vi "Feeder_Begin.vi"   [LabVIEW 2020]
uses:
  Subsystems/Magazine/Magazine_Cluster.ctl
  Subsystems/Magazine/Magazine_Control_States.ctl
  Subsystems/Intake/Intake_cluster.ctl
  Subsystems/Intake/Intake_control_states.ctl
  Subsystems/Funnel/Funnel_Cluster.ctl
  Subsystems/Funnel/Control_States_Funnel.ctl
  Feeder_Cluster.ctl
  Feeder_Control_States.ctl
  Globals/Magazine_Globals.vi
  Globals/Intake_Globals.vi
  Globals/Funnel_global.vi
  Globals/Feeder_Globals.vi
types:
  T1 = typedef "Feeder_Cluster.ctl" = cluster{"Firing":bool, "Load":bool, "Magazine_%Vbus":dbl, "Funnel_%Vbus":dbl, "Intake_%Vbus":dbl, "Manual_Extend":bool, "Outtake":bool, "Parameters":dbl[], "Auto_Notifier":refnum<notifier>, "Step":i32, "Control_States":T2}
  T2 = typedef "Feeder_Control_States.ctl" = enum16{"No-Op", "Manual", "Load", "Outtake", "Firing", "Test", "Command_Feed", "Command_Shoot"}
  T3 = typedef "Funnel_Cluster.ctl" = cluster{"Control States":T4, "%Vbus":dbl}
  T4 = typedef "Control_States_Funnel.ctl" = enum16{"No_Op", "Manual_Op", "Load", "Firing", "Outtake"}
  T5 = typedef "Intake_cluster.ctl" = cluster{"control_states":T6, "%Vbus":dbl, "Trigger?":bool, "Manual_Extend?":bool, "Auto_Notifier":refnum<notifier>, "Step":dbl, "Parameter 1":dbl, "Parameter 2":dbl, "Parameter 3":dbl}
  T6 = typedef "Intake_control_states.ctl" = enum16{"No_Op", "Intake", "Manual", "Outtake", "Extend_No_Motor", "Retract_No_Motor"}
  T7 = typedef "Magazine_Cluster.ctl" = cluster{"Control_States":T8, "%Vbus":dbl, "Load_Magazine":bool, "Firing_Magazine":bool, "Velocity":dbl}
  T8 = typedef "Magazine_Control_States.ctl" = enum16{"No-Op", "Manual_%Vbus", "Manual_Speed_Control", "Test_Speed_Control", "Load", "Firing", "Outtake"}
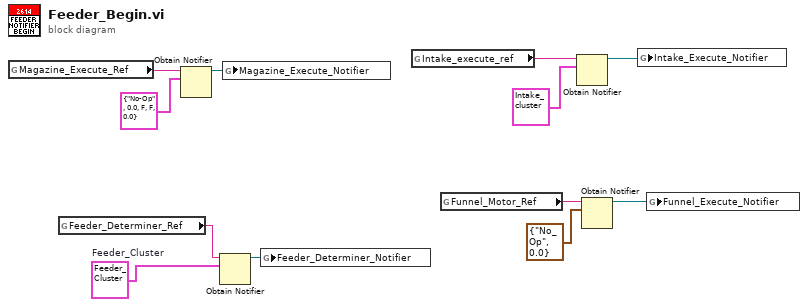
[diagram p0: block diagram]
diagram:
  w2 = T1 {"Firing"=FALSE, "Load"=FALSE, "Magazine_%Vbus"=0.0, "Funnel_%Vbus"=0.0, "Intake_%Vbus"=0.0, "Manual_Extend"=FALSE, "Outtake"=FALSE, "Parameters"=[], "Auto_Notifier"=refnum, "Step"=0, "Control_States"=enum."No-Op"}  # Feeder_Cluster
  n1 = global read "Magazine_Globals.vi" "Magazine_Execute_Ref"() -> (w11:string)
  n2 = global read "Feeder_Globals.vi" "Feeder_Determiner_Ref"() -> (w3:string)
  n3 = Obtain Notifier(name (unnamed)=w11, notification data type=T7 {"Control_States"=enum."No-Op", "%Vbus"=0.0, "Load_Magazine"=FALSE, "Firing_Magazine"=FALSE, "Velocity"=0.0}) -> (notifier out=w12:refnum<notifier>)  [unwired: 2 in, 2 out]
  n4 = Obtain Notifier(name (unnamed)=w3, notification data type=w2) -> (notifier out=w1:refnum<notifier>)  [unwired: 2 in, 2 out]
  n5 = global write "Magazine_Globals.vi" "Magazine_Execute_Notifier"(w12) -> ()
  n6 = global write "Feeder_Globals.vi" "Feeder_Determiner_Notifier"(w1) -> ()
  n7 = global read "Intake_Globals.vi" "Intake_execute_ref"() -> (w8:string)
  n8 = global read "Funnel_global.vi" "Funnel_Motor_Ref"() -> (w4:string)
  n9 = Obtain Notifier(name (unnamed)=w8, notification data type=T5 {"control_states"=enum."Intake", "%Vbus"=0.0, "Trigger?"=FALSE, "Manual_Extend?"=FALSE, "Auto_Notifier"=refnum, "Step"=0.0, "Parameter 1"=0.0, "Parameter 2"=0.0, "Parameter 3"=0.0}) -> (notifier out=w9:refnum<notifier>)  [unwired: 2 in, 2 out]
  n10 = Obtain Notifier(name (unnamed)=w4, notification data type=T3 {"Control States"=enum."No_Op", "%Vbus"=0.0}) -> (notifier out=w6:refnum<notifier>)  [unwired: 2 in, 2 out]
  n11 = global write "Intake_Globals.vi" "Intake_Execute_Notifier"(w9) -> ()
  n12 = global write "Funnel_global.vi" "Funnel_Execute_Notifier"(w6) -> ()
